vi "continuous_ramp_rev1.vi"() -> ()   [LabVIEW 2018]
uses:
  <vilib>/myRIO/Instrument Drivers/Onboard IO/DIO/typedefs/DIO Reference.ctl
  <vilib>/myRIO/Common/Instrument Driver Framework/Utilities/typedefs/myRIO Generic Hardware Reference.ctl
  <vilib>/myRIO/Common/Instrument Driver Framework/Utilities/typedefs/Hardware Version Enum.ctl
  <vilib>/myRIO/Common/Instrument Driver Framework/Utilities/typedefs/myRIO v1.0 Reference.ctl
  <vilib>/myRIO/Common/Instrument Driver Framework/Utilities/typedefs/Generic FPGA Reference.ctl
  <vilib>/myRIO/Common/Instrument Driver Framework/myRIO v1.0/DIO/typedefs/DIO Channels List.ctl
  <vilib>/myRIO/Common/Instrument Driver Framework/myRIO v1.0/DIO/typedefs/DIO Channels Enum.ctl
  <vilib>/userdefined/High Color/nirio_resource_hc.ctl
  <vilib>/myRIO/Instrument Drivers/Onboard IO/AI/typedefs/AI Reference.ctl
  <vilib>/myRIO/Common/Instrument Driver Framework/myRIO v1.0/AI/typedefs/AI Channels List.ctl
  <vilib>/myRIO/Common/Instrument Driver Framework/myRIO v1.0/AI/typedefs/AI Channels Enum.ctl
  <vilib>/myRIO/Common/Instrument Driver Framework/Utilities/typedefs/Analog Scaling Constants List.ctl
  <vilib>/myRIO/Common/Instrument Driver Framework/Utilities/typedefs/Analog Scaling Constants.ctl
  <vilib>/myRIO/Instrument Drivers/Onboard IO/AO/typedefs/AO Reference.ctl
  <vilib>/myRIO/Common/Instrument Driver Framework/myRIO v1.0/AO/typedefs/AO Channels List.ctl
  <vilib>/myRIO/Common/Instrument Driver Framework/myRIO v1.0/AO/typedefs/AO Channels Enum.ctl
  <vilib>/myRIO/Common/Instrument Driver Framework/myRIO v1.0/AO/vis/myRIO v1.1 Open AO.vi
  <vilib>/myRIO/Common/Instrument Driver Framework/myRIO v1.0/AI/vis/myRIO v1.1 Open AI.vi
  <vilib>/myRIO/Common/Instrument Driver Framework/myRIO v1.0/DIO/vis/myRIO v1.1 Open DIO.vi
  <vilib>/myRIO/Common/Instrument Driver Framework/Utilities/vis/Validate Channels.vi
  <vilib>/myRIO/Common/Instrument Driver Framework/myRIO v1.0/AO/vis/myRIO v1.0 Reserve AO.vi
  <vilib>/myRIO/Common/Instrument Driver Framework/myRIO v1.0/AI/vis/myRIO v1.0 Reserve AI.vi
  <vilib>/myRIO/Common/Instrument Driver Framework/myRIO v1.0/DIO/vis/myRIO v1.0 Reserve DIO.vi
  <vilib>/myRIO/Common/Instrument Driver Framework/myRIO v1.0/DIO/vis/myRIO v1.0 Close DIO.vi
  <vilib>/myRIO/Common/Instrument Driver Framework/myRIO v1.0/AI/vis/myRIO v1.0 Close AI.vi
  <vilib>/myRIO/Common/Instrument Driver Framework/myRIO v1.0/AO/vis/myRIO v1.0 Close AO.vi
  <vilib>/myRIO/Common/Instrument Driver Framework/myRIO v1.0/AO/vis/myRIO v1.0 Build MUX Configuration AO.vi
  <vilib>/myRIO/Common/Instrument Driver Framework/myRIO v1.0/Resource Manager/vis/myRIO v1.0 Reserve Channel List.vi
  <vilib>/myRIO/Common/Instrument Driver Framework/myRIO v1.0/AI/vis/myRIO v1.0 Build MUX Configuration AI.vi
  <vilib>/myRIO/Common/Instrument Driver Framework/myRIO v1.0/DIO/vis/myRIO v1.0 Build MUX Configuration DIO.vi
  <vilib>/myRIO/Common/Instrument Driver Framework/myRIO v1.0/DIO/vis/myRIO v1.0 Unreserve DIO.vi
  <vilib>/myRIO/Common/Instrument Driver Framework/myRIO v1.0/AI/vis/myRIO v1.0 Unreserve AI.vi
  <vilib>/myRIO/Common/Instrument Driver Framework/myRIO v1.0/AO/vis/myRIO v1.0 Unreserve AO.vi
  <vilib>/myRIO/Common/Instrument Driver Framework/myRIO v1.0/Resource Manager/vis/myRIO v1.0 Reserve Channel.vi
  <vilib>/myRIO/Common/Instrument Driver Framework/myRIO v1.0/Resource Manager/vis/myRIO v1.0 Unreserve Channel.vi
  <vilib>/myRIO/Common/Instrument Driver Framework/myRIO v1.0/Resource Manager/vis/myRIO v1.0 Create Configuration List.vi
  <vilib>/myRIO/Common/Instrument Driver Framework/myRIO v1.0/Resource Manager/vis/myRIO v1.0 Unreserve Channel List.vi
  <vilib>/myRIO/Common/Instrument Driver Framework/myRIO v1.0/Resource Manager/vis/myRIO v1.0 Build Mutex Name.vi
  <vilib>/Utility/VariantDataType/GetNumericInfo.vi
  <vilib>/Utility/error.llb/Error Cluster From Error Code.vi
  <vilib>/myRIO/Common/Instrument Driver Framework/myRIO v1.0/myRIO v1.1 Open.vi
  <vilib>/myRIO/Common/Instrument Driver Framework/Utilities/vis/IO Manager.vi
  <vilib>/myRIO/Common/Instrument Driver Framework/Utilities/vis/Configuration Manager.vi
  <vilib>/myRIO/Common/Instrument Driver Framework/myRIO v1.0/Resource Manager/vis/myRIO v1.0 Configure IO.vi
  <vilib>/myRIO/Common/Instrument Driver Framework/myRIO v1.0/myRIO v1.0 Close.vi
  <vilib>/myRIO/Common/Instrument Driver Framework/myRIO v1.0/DIO/vis/myRIO v1.0 Write DIO.vi
  <vilib>/myRIO/Common/Instrument Driver Framework/myRIO v1.0/AI/vis/myRIO v1.0 Get Scaling Constants AI.vi
  <vilib>/myRIO/Common/Instrument Driver Framework/myRIO v1.0/AO/vis/myRIO v1.0 Get Scaling Constants AO.vi
  <vilib>/myRIO/Common/Instrument Driver Framework/myRIO v1.0/AO/vis/myRIO v1.0 Write AO.vi
  <vilib>/myRIO/Common/Instrument Driver Framework/myRIO v1.0/AI/vis/myRIO v1.0 Read AI.vi
  <vilib>/myRIO/Common/Instrument Driver Framework/myRIO v1.0/DIO/vis/myRIO v1.0 Shutdown DIO.vi
  <vilib>/myRIO/Instrument Drivers/Onboard IO/DIO/vis/myRIO DIO Open.xnode
  <vilib>/myRIO/Instrument Drivers/Onboard IO/AI/vis/myRIO AI Open.xnode
  <vilib>/myRIO/Instrument Drivers/Onboard IO/AO/vis/myRIO AO Open.xnode
  <vilib>/myRIO/Instrument Drivers/Onboard IO/AO/AO.lvlib
  <vilib>/myRIO/Instrument Drivers/Onboard IO/DIO/DIO.lvlib
  <vilib>/myRIO/Instrument Drivers/Onboard IO/AI/AI.lvlib
  <vilib>/Analysis/NI_AAL_SigProc.lvlib
panel:
  out "loop rate":u32
  out "XY Graph":cluster{"Y":dbl[], "Y":dbl[]}[](graph)
  out "Approx. Corrected \nThickness (um)":dbl
  in  "Tab Control":T1(tab)
  in  "Vmax":dbl=2.6
  in  "Vmin":dbl=1.5
  in  "No. data points":i32=2500
  in  "sampling delay":u32=1
  in  "peak threshold":dbl=1.6 format="%#_13g"
  in  "width":i32=50
  in  "Confocal":tag[](array[tag])=["A/AI0"]
  in  "VC amp enable":tag[](array[tag])=["A/DIO0"]
  in  "VC  2":tag[](array[tag])=["A/AO0"]
  in  "cap probe":tag[](array[tag])
  in  "take data":bool
  in  "stop":bool
  out "Uncorrected \nThickness (um)":dbl
  out "Cap peak 2 (um)":dbl
  out "Cap peak 1 (um)":dbl
  out "XY Graph 2":cluster{"Y":dbl[], "Y":dbl[]}[](graph)
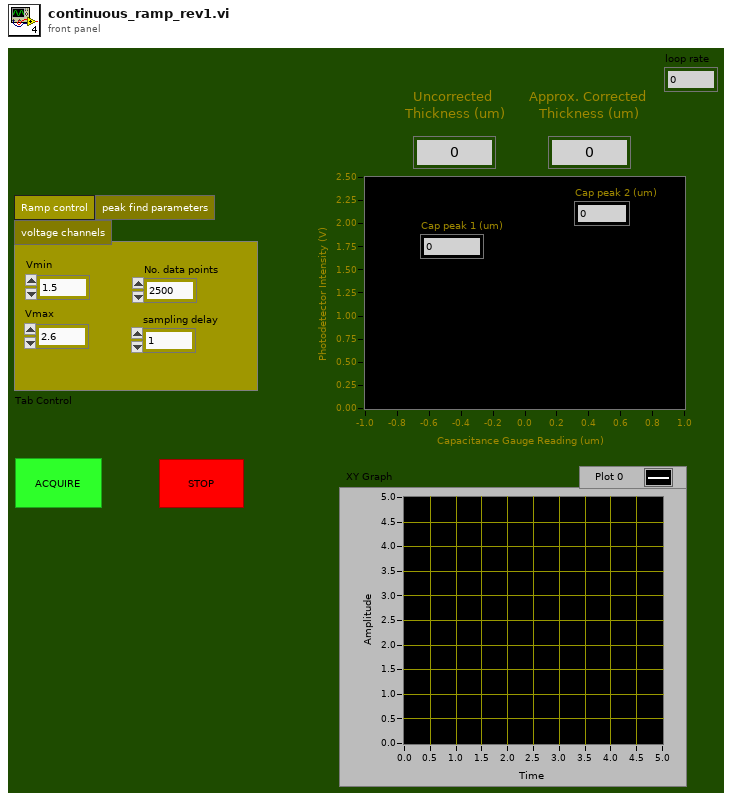
[diagram p1: front panel]
types:
  T1 = enum32{"Ramp control", "peak find parameters", "voltage channels"}
  T2 = enum16{"initialize", "ramp up", "max", "ramp down", "min"}
  T3 = typedef "nirio_resource_hc.ctl" = tag
  T4 = typedef "Hardware Version Enum.ctl" = enum16{"Unknown", "myRIO-1900", "myRIO-1950", "roboRIO", "NI ELVIS RIO CM", "ELVIS III"}
  T5 = typedef "AO.lvlib/AO Reference.ctl" = cluster{"myRIO Reference":T6, "AO Channel List":T9, "AO Scaling Constant List":T11}
  T6 = typedef "myRIO Generic Hardware Reference.ctl" = cluster{"myRIO Model":T4, "myRIO Hardware Reference":T7}
  T7 = typedef "myRIO v1.0 Reference.ctl" = cluster{"Generic FPGA Reference":T8, "Allow multiple opens":bool}
  T8 = typedef "Generic FPGA Reference.ctl" = refnum<k20>
  T9 = typedef "AO Channels List.ctl" = T10[]
  T10 = typedef "AO Channels Enum.ctl" = enum16{"Not Connected", "AudioOut/Left", "AudioOut/Right", "C/AO0", "C/AO1", "A/AO0", "A/AO1", "B/AO0", "B/AO1"}
  T11 = typedef "Analog Scaling Constants List.ctl" = T12[]
  T12 = typedef "Analog Scaling Constants.ctl" = cluster{"LSB Weight (Volts)":dbl, "Offset (Volts)":dbl, "Signed?":bool}
  T13 = typedef "DIO.lvlib/DIO Reference.ctl" = cluster{"myRIO Reference":T6, "DIO Channels List":T14}
  T14 = typedef "DIO Channels List.ctl" = T15[]
  T15 = typedef "DIO Channels Enum.ctl" = enum16{"Not Connected", "C/DIO0", "C/DIO1", "C/DIO2", "C/DIO3", "C/DIO4", "C/DIO5", "C/DIO6", "C/DIO7", "A/DIO0", "A/DIO1", "A/DIO2", "A/DIO3", "A/DIO4", "A/DIO5", "A/DIO6", "A/DIO7", "A/DIO8", "A/DIO9", "A/DIO10", "A/DIO11", "A/DIO12", "A/DIO13", "A/DIO14", "A/DIO15", "A/DIO16", "A/DIO17", "A/DIO18", "A/DIO19", "B/DIO0", "B/DIO1", "B/DIO2", "B/DIO3", "B/DIO4", "B/DIO5", "B/DIO6", "B/DIO7", "B/DIO8", "B/DIO9", "B/DIO10", "B/DIO11", "B/DIO12", "B/DIO13", "B/DIO14", "B/DIO15", "B/DIO16", "B/DIO17", "B/DIO18", "B/DIO19", "LED0", "LED1", "LED2", "LED3", "Button0", "DIO/DIO0", "DIO/DIO1", "DIO/DIO2", "DIO/DIO3", "DIO/DIO4", "DIO/DIO5", "DIO/DIO6", "DIO/DIO7", "DIO/DIO8", "DIO/DIO9", "SPI/CS0", "SPI/CS1", "SPI/CS2", "SPI/CS3", "LED RADIO (Green)", "LED RADIO (Red)", "LED COMM (Green)", "LED COMM (Red)", "LED MODE (Green)", "LED MODE (Red)"}
  T16 = typedef "AI.lvlib/AI Reference.ctl" = cluster{"myRIO Reference":T6, "AI Channels List":T17, "AI Scaling Constants List":T11}
  T17 = typedef "AI Channels List.ctl" = T18[]
  T18 = typedef "AI Channels Enum.ctl" = enum16{"Not Connected", "AudioIn/Left", "AudioIn/Right", "C/AI0", "C/AI1", "A/AI0", "A/AI1", "A/AI2", "A/AI3", "A/AI4", "A/AI5", "A/AI6", "A/AI7", "B/AI0", "B/AI1", "B/AI2", "B/AI3", "B/AI4", "B/AI5", "B/AI6", "B/AI7", "AI/AI0", "AI/AI1", "AI/AI2", "AI/AI3", "A/AI0 (DIFF)", "A/AI1 (DIFF)", "A/AI2 (DIFF)", "A/AI3 (DIFF)", "B/AI0 (DIFF)", "B/AI1 (DIFF)", "B/AI2 (DIFF)", "B/AI3 (DIFF)"}
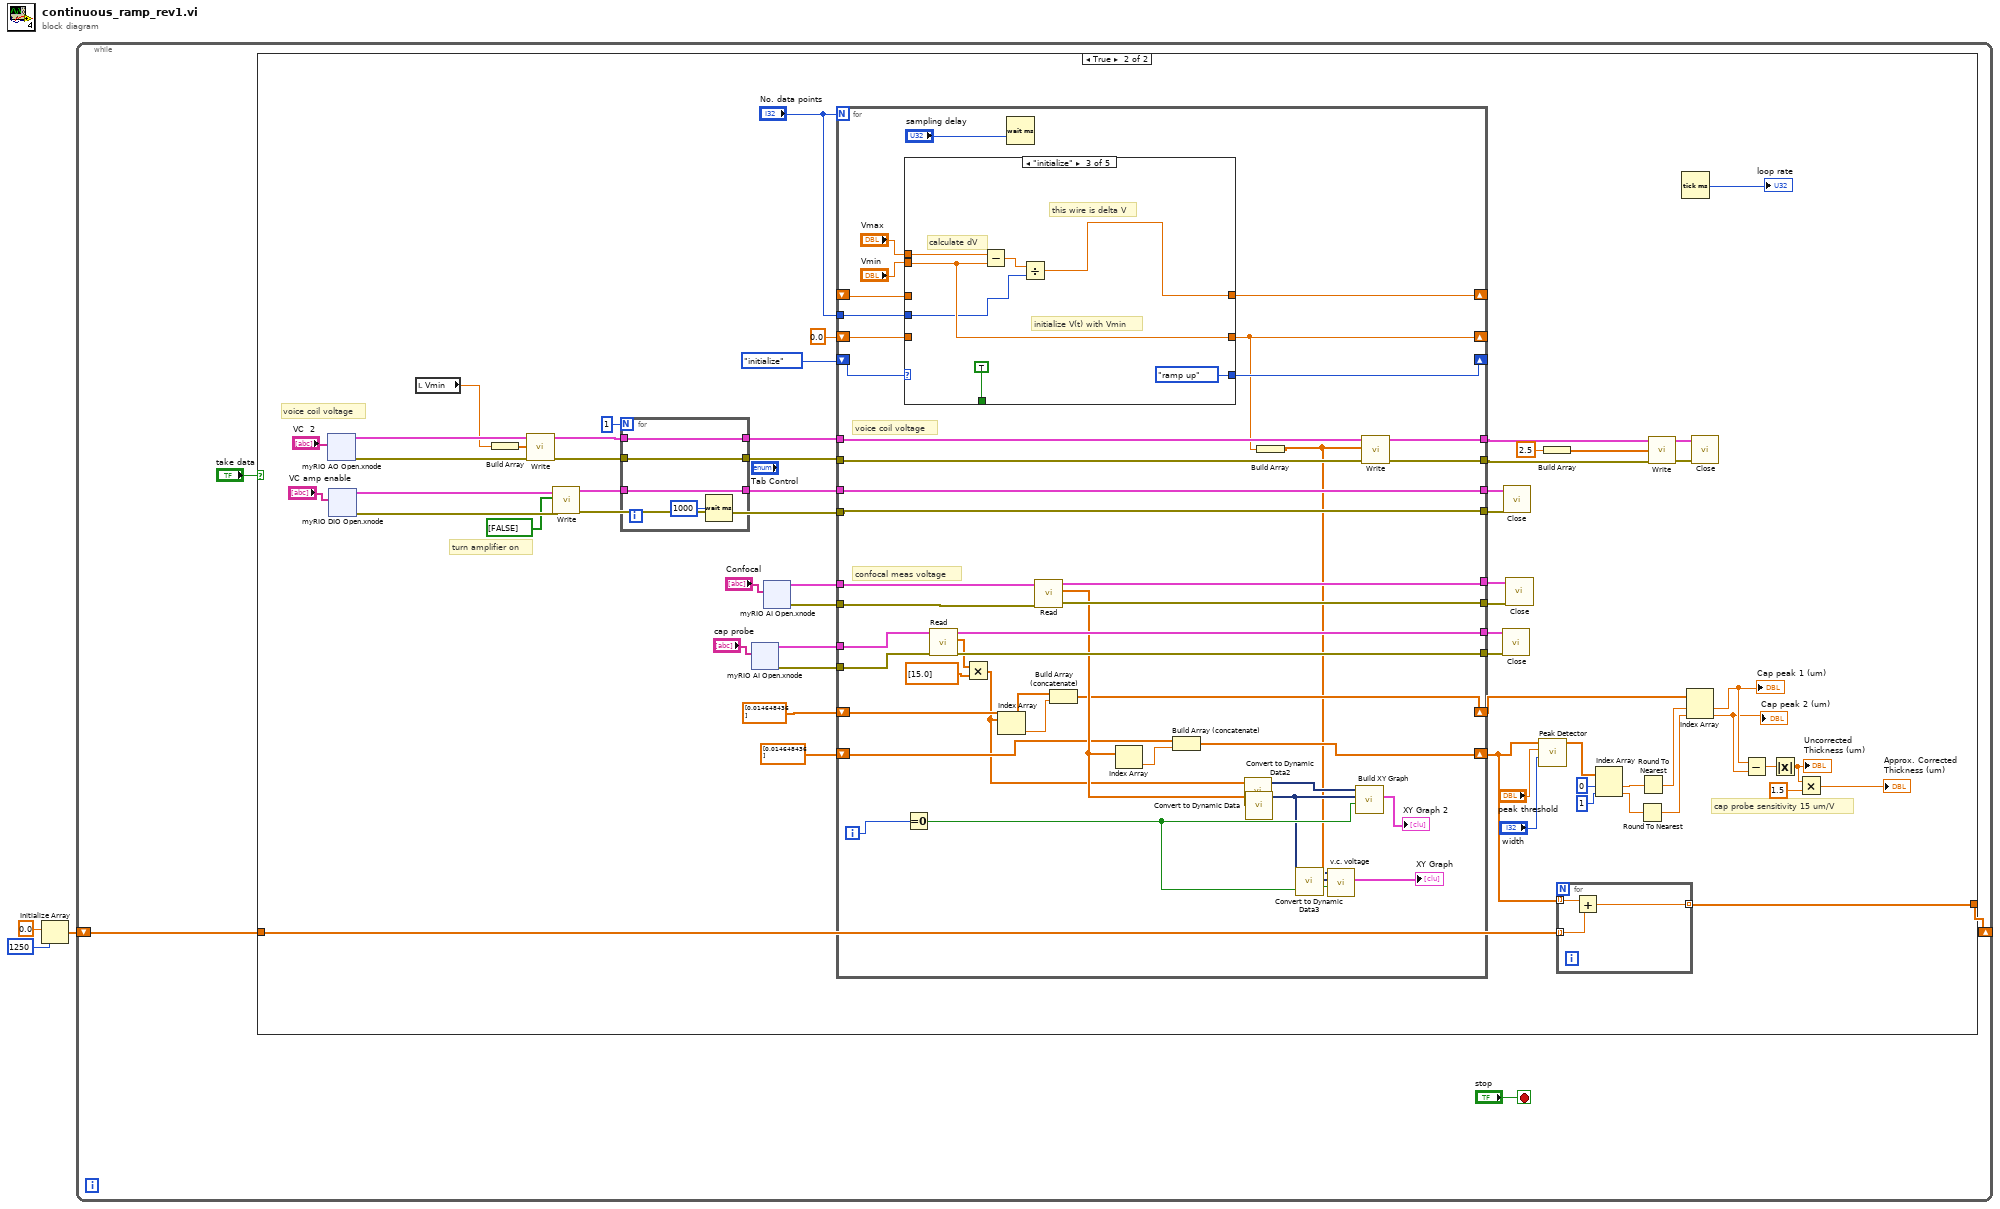
[diagram p0: block diagram]
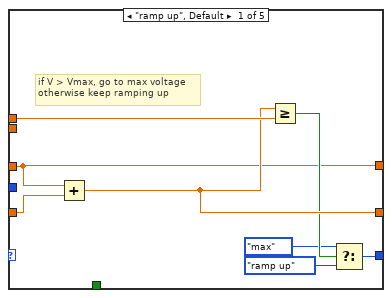
[diagram p3: hidden frame]
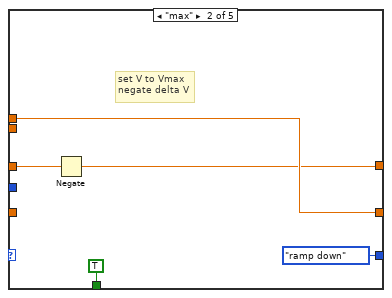
[diagram p4: hidden frame]
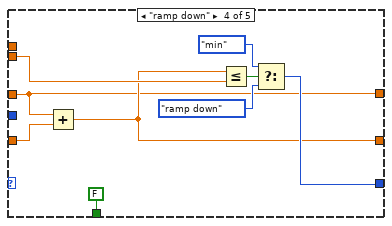
[diagram p5: hidden frame]
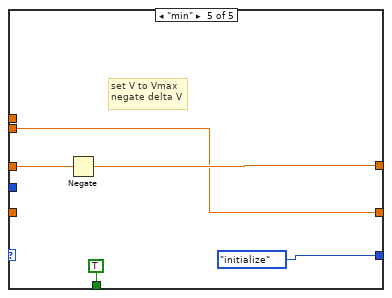
[diagram p6: hidden frame]
diagram:
  n1 = Initialize Array(0.0 ("element"), 1250 ("dimension size")) -> (w1:dbl[])
  n2 = while {
    shift-right: [w4] -> _
    shift-left: w1 -> [w5]
    stop <- "stop" stop-if-true
    n3 = case shown="True" "take data" {
      tunnel: w5 -> [w8 w15]
      tunnel: [w8 w14] -> w4
      frame False {
      }
      frame True {
        # "turn amplifier on"
        # "voice coil voltage"
        # "cap probe sensitivity 15 um/V"
        n4 = xnode "myRIO AO Open.xnode"("Channel Names"="VC  2") -> ("error out"=w45:errorcluster, "AO Ref Out"=w46:T5)  [unwired: 2 in]
        n5 = xnode "myRIO DIO Open.xnode"("Channel Names"="VC amp enable") -> ("error out"=w44:errorcluster, "DIO Ref Out"=w43:T13)  [unwired: 2 in]
        n6 = local read "Vmin"() -> (w17:dbl)
        n7 = Build Array(w17) -> (w47:dbl[])
        n8 = call <vilib>:"Write.vi"("error in (no error)"=w45, "Values"=w47, "AO Ref In"=w46) -> ("error out"=w29:errorcluster, "AO Ref Out"=w33:T5)  [unwired: 6 in]
        n9 = call <vilib>:"Write.vi"("error in (no error)"=w44, "Values"=bool[] [FALSE], "DIO Ref In"=w43) -> ("error out"=w41:errorcluster, "DIO Ref Out"=w31:T13)  [unwired: 6 in]
        n10 = for {
          N: 1 -> [_]
          tunnel: w33 -> [w75]
          tunnel: [w75] -> w32
          tunnel: w31 -> [w74]
          tunnel: [w74] -> w30
          tunnel: w29 -> [w73]
          tunnel: [w73] -> w28
          n11 = Wait (ms)(milliseconds to wait=u32 1000) -> ()  [unwired: 1 out]
        }
        n12 = xnode "myRIO AI Open.xnode"("Channel Names"="cap probe") -> ("error out"=w58:errorcluster, "AI Ref Out"=w59:T16)  [unwired: 2 in]
        n13 = xnode "myRIO AI Open.xnode"("Channel Names"="Confocal") -> ("error out"=w61:errorcluster, "AI Ref Out"=w64:T16)  [unwired: 2 in]
        n14 = for {
          N: "No. data points" -> [_]
          shift-right: [w84] -> _
          shift-left: 0.0 ("V") -> [w114]
          shift-right: [w115] -> _
          shift-left: _ -> [w113]
          shift-right: [w111] -> _
          shift-left: T2."initialize" -> [w112]
          tunnel: w32 -> [w109]
          tunnel: w28 -> [w110]
          tunnel: [w108] -> w38
          tunnel: [w107] -> w37
          tunnel: w64 -> [w106]
          tunnel: [w105] -> w63
          tunnel: [w104] -> w62
          tunnel: w61 -> [w103]
          tunnel: w59 -> [w101]
          tunnel: w58 -> [w100]
          tunnel: [w99] -> w57
          tunnel: [w98] -> w56
          shift-right: [w91] -> w16
          shift-left: dbl[] [0.014648436] ("Values") -> [w95]
          shift-right: [w92] -> w52
          shift-left: dbl[] [0.014648436] ("Values") -> [w94]
          tunnel: w30 -> [w90]
          tunnel: [w90] -> w26
          tunnel: w41 -> [w89]
          tunnel: [w89] -> w27
          tunnel: "No. data points" -> [w83]
          i -> [w85]
          # "confocal meas voltage"
          # "voice coil voltage"
          n15 = case shown="\"initialize\"" w112 {
            tunnel: "Vmin" -> [_ _ w136 w144 w149]
            tunnel: "Vmax" -> [w124 w130 w137 _ _]
            tunnel: [w118 w128 w132 w139 w150] -> w115
            tunnel: [w123 w130 w136 w140 w149] -> w84
            tunnel: w114 -> [w125 _ _ w145 _]
            tunnel: w113 -> [w118 w129 _ w139 w151]
            tunnel: [w119 T2."ramp down" T2."ramp up" w141 T2."initialize"] -> w111
            tunnel: [_ TRUE TRUE FALSE TRUE] -> _
            tunnel: w83 -> [_ _ w131 _ _]
            frame "ramp up", Default {
              # "if V > Vmax, go to max voltage\notherwise keep ramping up"
              n16 = Add(x=w118, y=w125) -> (x+y=w123:dbl)
              n17 = Greater Or Equal?(x=w123, y=w124) -> (x >= y?=w122:bool)
              n18 = Select(t=T2."max", s=w122, f=T2."ramp up") -> (s? t:f=w119:T2)
            }
            frame "max" {
              # "set V to Vmax\nnegate delta V"
              n19 = Negate(x=w129) -> (-x=w128:dbl)
            }
            frame "initialize" {
              # "calculate dV"
              # "initialize V(t) with Vmin"
              # "this wire is delta V"
              n20 = Subtract(x=w137, y=w136) -> (x-y=w133:dbl)
              n21 = Divide(x=w133, y=w131) -> (x/y=w132:dbl)
            }
            frame "ramp down" {
              n22 = Add(x=w139, y=w145) -> (x+y=w140:dbl)
              n23 = Less Or Equal?(x=w140, y=w144) -> (x <= y?=w146:bool)
              n24 = Select(t=T2."min", s=w146, f=T2."ramp down") -> (s? t:f=w141:T2)
            }
            frame "min" {
              # "set V to Vmax\nnegate delta V"
              n25 = Negate(x=w151) -> (-x=w150:dbl)
            }
          }
          n26 = Equal To 0?(x=w85) -> (x = 0?=w79:bool)
          n27 = call <vilib>:"Read.vi"("error in (no error)"=w100, "AI Ref In"=w101) -> ("error out"=w98:errorcluster, "Values"=w88:dbl[], "AI Ref Out"=w99:T16)  [unwired: 7 in]
          n28 = Multiply(x=w88, y=dbl[] [15.0]) -> (x*y=w86:dbl[])
          n29 = Index Array(array=w86) -> (element=w93:dbl)  [unwired: 1 in]
          n30 = Wait (ms)(milliseconds to wait="sampling delay") -> ()  [unwired: 1 out]
          n31 = call <vilib>:"Read.vi"("error in (no error)"=w103, "AI Ref In"=w106) -> ("error out"=w104:errorcluster, "Values"=w97:dbl[], "AI Ref Out"=w105:T16)  [unwired: 7 in]
          n32 = Build Array (concatenate)(w94, w93) -> (w92:dbl[])
          n33 = Index Array(array=w97) -> (element=w96:dbl)  [unwired: 1 in]
          n34 = Build Array (concatenate)(w95, w96) -> (w91:dbl[])
          n35 = call "Convert to Dynamic Data2"("Array"=w86) -> ("Dynamic Data Type"=w80:dynamicdata)  [unwired: 3 in]
          n36 = call "Convert to Dynamic Data"("Array"=w97) -> ("Dynamic Data Type"=w78:dynamicdata)  [unwired: 3 in]
          n37 = Build Array(w84) -> (w77:dbl[])
          n38 = call "Convert to Dynamic Data3"("Array"=w77) -> ("Dynamic Data Type"=w76:dynamicdata)  [unwired: 3 in]
          n39 = call "v.c. voltage"("Reset"=w79, "Y Input"=w78, "X Input"=w76) -> ("XY Graph"=→"XY Graph":cluster{"X":dbl[], "Y":dbl[]}[])  [unwired: 7 in, 1 out]
          n40 = call "Build XY Graph"("Reset"=w79, "Y Input"=w78, "X Input"=w80) -> ("XY Graph"=→"XY Graph 2":cluster{"X":dbl[], "Y":dbl[]}[])  [unwired: 7 in, 1 out]
          n41 = call <vilib>:"Write.vi"("error in (no error)"=w110, "Values"=w77, "AO Ref In"=w109) -> ("error out"=w107:errorcluster, "AO Ref Out"=w108:T5)  [unwired: 6 in]
        }
        n42 = call <vilib>:"Close.vi"("error in (no error)"=w56, "AI Ref In"=w57) -> ()  [unwired: 9 in, 1 out]
        n43 = call <vilib>:"Close.vi"("error in (no error)"=w27, "DIO Ref In"=w26) -> ()  [unwired: 9 in, 1 out]
        n44 = call <vilib>:"Close.vi"("error in (no error)"=w62, "AI Ref In"=w63) -> ()  [unwired: 9 in, 1 out]
        n45 = call <vilib>:"Peak Detector.vi"("width"="width", "threshold"="peak threshold", "X"=w16) -> ("Locations"=w21:dbl[])  [unwired: 4 in, 4 out]
        n46 = Build Array(2.5 ("element")) -> (w40:dbl[])
        n47 = for {
          tunnel: w16 -> [w71] mode=indexing
          tunnel: w15 -> [w70] mode=indexing
          tunnel: [w69] -> w14 mode=indexing
          n48 = Add(x=w71, y=w70) -> (x+y=w69:dbl)
        }
        n49 = Index Array(array=w21, index #1=0 ("index"), index #2=1 ("index")) -> (element #1=w22:dbl, element #2=w20:dbl)
        n50 = Round To Nearest(number=w20) -> (nearest integer value=w18:dbl)
        n51 = Round To Nearest(number=w22) -> (nearest integer value=w19:dbl)
        n52 = call <vilib>:"Write.vi"("error in (no error)"=w37, "Values"=w40, "AO Ref In"=w38) -> ("error out"=w35:errorcluster, "AO Ref Out"=w36:T5)  [unwired: 6 in]
        n53 = Tick Count (ms)() -> (millisecond timer value=→"loop rate":u32)
        n54 = Index Array(array=w52, index #1=w19, index #2=w18) -> (element #1=w51:dbl, element #2=w50:dbl)
        "Cap peak 1 (um)" <- w51
        "Cap peak 2 (um)" <- w50
        n55 = call <vilib>:"Close.vi"("error in (no error)"=w35, "AO Ref In"=w36) -> ()  [unwired: 9 in, 1 out]
        n56 = Subtract(x=w51, y=w50) -> (x-y=w49:dbl)
        n57 = Absolute Value(x=w49) -> (abs(x)=w12:dbl)
        "Uncorrected \nThickness (um)" <- w12
        n58 = Multiply(x=w12, y=1.5) -> (x*y=→"Approx. Corrected \nThickness (um)":dbl)
      }
    }
  }
